vi "Read Data (String).vi"(8 "error in (no error)":errorcluster, 11 "Handle":u32) -> (0 "error out":errorcluster, 1 "Bytes Read":u32, 2 "Read Buffer":string, 3 "Handle out":u32)   [LabVIEW 2019, in "D2XX-lv.lvlib"]
doc: "Read string data from an open device."
uses:
  D2XX-lv.lvlib
  <instrlib>/FTDI/D2XX/D2XX.lvlib
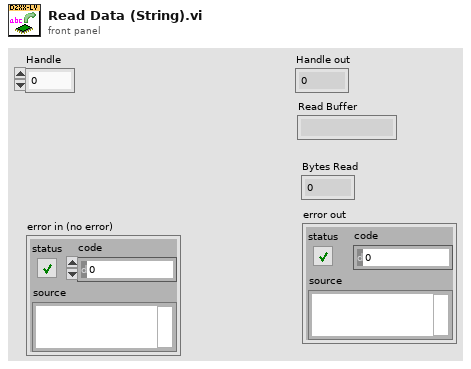
[diagram p1: front panel]
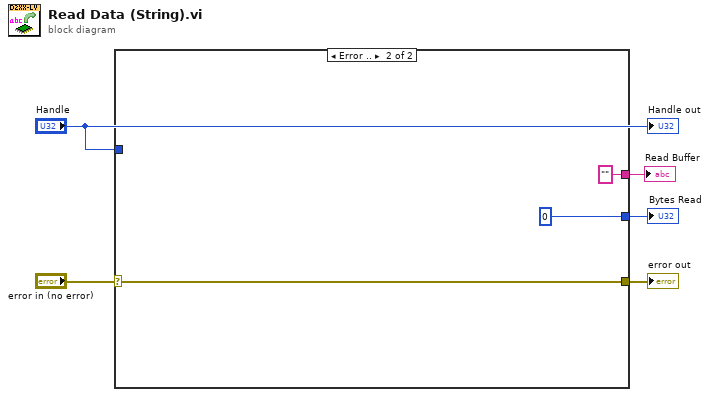
[diagram p0: block diagram]
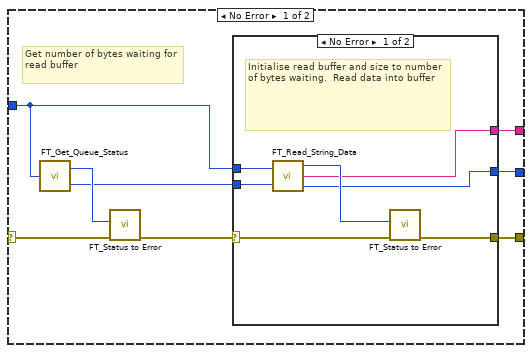
[diagram p2: hidden frame]
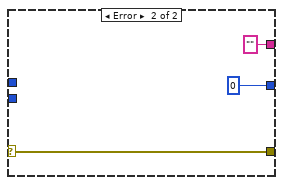
[diagram p3: hidden frame]
diagram:
  n1 = case shown="Error .." "error in (no error)" {
    selector: "error in (no error)" -> [w13 w26]
    tunnel: [w10 w26] -> w4
    tunnel: "Handle" -> [w9 _]
    tunnel: [w7 u32 0 ("Bytes Written")] -> w3
    tunnel: [w6 "" ("Read Data")] -> w1
    frame No Error {
      # "Get number of bytes waiting for read buffer"
      n2 = call <instrlib>:"FT_Get_Queue_Status.vi"("Handle"=w9) -> ("FT_Status"=w12:u32, "Bytes Waiting"=w8:u32)
      n3 = call "FT_Status to Error.vi"("error in (no error)"=w13, "FT_Status"=w12) -> ("error out"=w11:errorcluster)  [unwired: 9 in]
      n4 = case shown="No Error" w11 {
        selector: w11 -> [w20 w23]
        tunnel: [w19 w23] -> w10
        tunnel: w9 -> [w17 _]
        tunnel: w8 -> [w18 _]
        tunnel: [w15 u32 0 ("Bytes Read")] -> w7
        tunnel: [w14 "" ("Read Data")] -> w6
        frame No Error {
          # "Initialise read buffer and size to number of bytes waiting.  Read data into buffer"
          n5 = call <instrlib>:"FT_Read_String_Data.vi"("Handle"=w17, "Bytes To Read"=w18) -> ("FT_Status"=w16:u32, "Read Data"=w14:string, "Bytes Read"=w15:u32)
          n6 = call "FT_Status to Error.vi"("error in (no error)"=w20, "FT_Status"=w16) -> ("error out"=w19:errorcluster)  [unwired: 9 in]
        }
        frame Error {
        }
      }
    }
    frame Error {
    }
  }
  "error out" <- w4
  "Bytes Read" <- w3
  "Read Buffer" <- w1
  "Handle out" <- "Handle"
